vi "Upload Segment.vi"(11 "Service Data Object in":refnum<class "Service Data Object.lvclass">) -> (1 "Request":refnum<class "CANopen Request Message.lvclass">, 2 "Expected Response":refnum<class "CANopen Response Message.lvclass">, 3 "Service Data Object out":refnum<class "Service Data Object.lvclass">)   [LabVIEW 2024, in "CANopen Master.lvlib" / "Service Data Object.lvclass"]
uses:
  Service Data Object.lvclass
  CANopen Request/CANopen Request Message.lvclass
  CANopen Response/CANopen Response Message.lvclass
  CANopen/FunctionCode.ctl
  Upload Segment Response Comparator/Upload Segment Response Comparator.lvclass
  Service Data Object.lvclass/Service Data Object.ctl
  SDO Response Compare Strategy/SDO Response Compare Strategy.lvclass/SDO Response Compare Strategy.ctl
  CANopen Master.lvlib
  CANopen Message/CANopen Message.lvclass
  SDO Response Compare Strategy/SDO Response Compare Strategy.lvclass
  D:/git/CANopen-XNET/SDO Response Compare Strategy/SDO Response Compare Strategy.lvclass
  D:/git/CANopen-XNET/Upload Segment Response Comparator/Upload Segment Response Comparator.lvclass
  D:/git/CANopen-XNET/CANopen Message/CANopen Message.lvclass
  D:/git/CANopen-XNET/CANopen Request/CANopen Request Message.lvclass
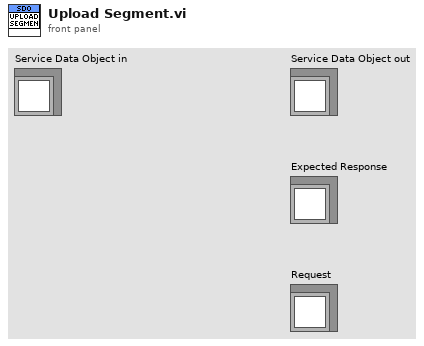
[diagram p1: front panel]
types:
  T1 = typedef "CANopen Master.lvlib/FunctionCode.ctl" = u16
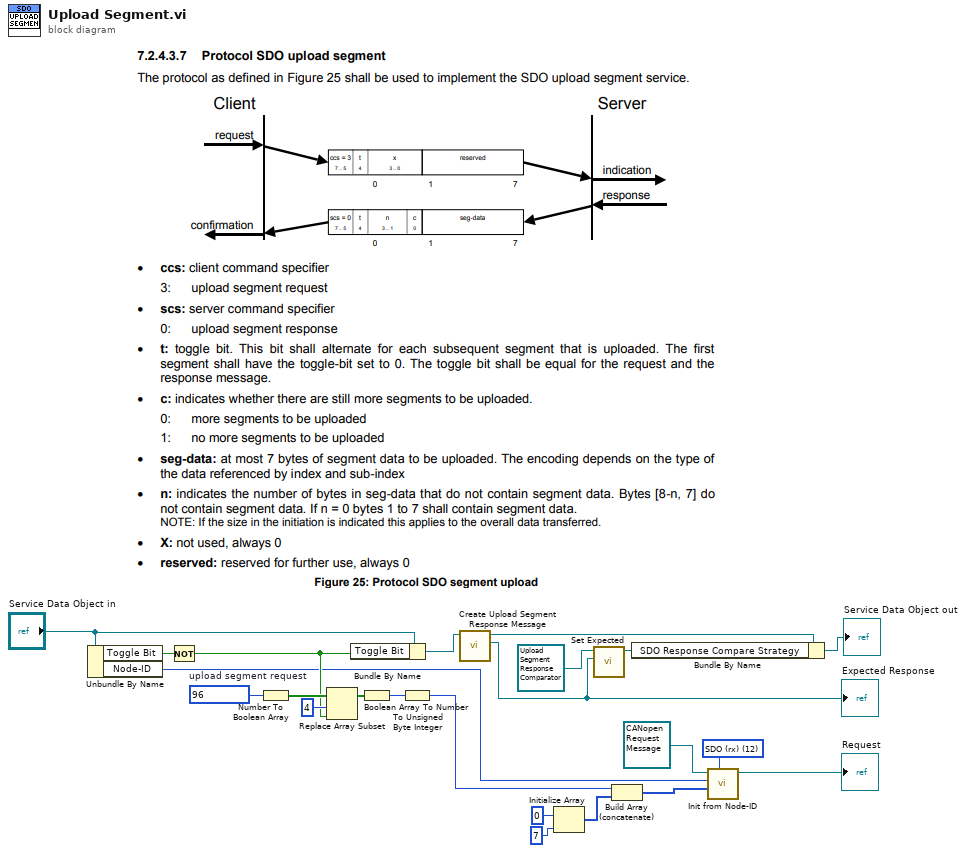
[diagram p0: block diagram]
diagram:
  w23 = T1 12 items=["EMCY"=1, "PDO1 (tx)"=3, "PDO1 (rx)"=4, "PDO2 (tx)"=5, "PDO2 (rx)"=6, "PDO3 (tx)"=7, "PDO3 (rx)"=8, "PDO4 (tx)"=9, "PDO4 (rx)"=10, "SDO (tx)"=11, "SDO (rx)"=12, "NMT error control"=14] ("Function code")
  w17 = u8 96  # upload segment request
  n1 = Unbundle By Name("Service Data Object in") -> ("Toggle Bit"=w18:bool, "Node-ID"=w4:u8)
  n2 = Not(x=w18) -> (.not. x?=w14:bool)
  n3 = Number To Boolean Array(number=w17) -> (Boolean array=w16:bool[])
  n4 = Replace Array Subset(array=w16, new element=w14, index=4) -> (w13:bool[])
  n5 = Bundle By Name(cluster="Service Data Object in", "Toggle Bit"=w14) -> (w19:refnum<class "Service Data Object.lvclass">)
  n6 = Boolean Array To Number(Boolean array=w13) -> (number=w12:u32)
  n7 = To Unsigned Byte Integer(number=w12) -> (unsigned 8bit integer=w11:u8)
  n8 = call "Create Upload Segment Response Message.vi"("Service Data Object in"=w19) -> ("Response Message"=w8:refnum<class "CANopen Response Message.lvclass">, "Service Data Object out"=w10:refnum<class "Service Data Object.lvclass">)  [unwired: 9 in]
  "Expected Response" <- w8
  n9 = Initialize Array(u8 0, 7 ("y")) -> (w1:u8[])
  n10 = call "Set Expected.vi"("CANopen Message"=w8, "SDO Response Compare Strategy in"=refnum<class "Upload Segment Response Comparator.lvclass"> refnum ("CANopen Master.lvlib:Upload Segment Response Comparator")) -> ("SDO Response Compare Strategy out"=w7:refnum<class "Upload Segment Response Comparator.lvclass">)  [unwired: 9 in]
  n11 = Build Array (concatenate)(w11, w1) -> (w22:u8[])
  n12 = Bundle By Name(cluster=w10, "SDO Response Compare Strategy"=w7) -> (→"Service Data Object out":refnum<class "Service Data Object.lvclass">)
  n13 = call "Init from Node-ID.vi"("Function code"=w23, "Data"=w22, "Node-ID"=w4, "CANopen Message in"=refnum<class "CANopen Request Message.lvclass"> refnum ("CANopen Master.lvlib:CANopen Request Message.lvclass")) -> ("CANopen Message out"=→"Request":refnum<class "CANopen Request Message.lvclass">)  [unwired: 7 in]
